vi "Pre Launch Init.vi"(11 "TopLevel in":refnum<class "TopLevel.lvclass">) -> (0 "error out":errorcluster, 3 "TopLevel out":refnum<class "TopLevel.lvclass">)   [LabVIEW 2019, in "TopLevel.lvlib" / "TopLevel.lvclass"]
doc: "(<B>Filename</B>: Actor Framework.lvlib:Actor.lvclass:Pre Launch Init.vi)\n\nDefines behavior that occurs after the Launch Nested Actor method is invoked but before the actor's Actor Core method begins running.\n\nBy default, this method does nothing. A descendant class may override it to define behavior."
uses:
  TopLevel.lvclass
  C:/Program Files/National Instruments/LabVIEW 2019/vi.lib/ActorFramework/Actor/Actor.lvclass
  TopLevel Messages/SendHistoryResults Msg/SendHistoryResults Msg.lvclass
  C:/Program Files/National Instruments/LabVIEW 2019/vi.lib/ActorFramework/Message/Message.lvclass
  Models/ImageResultModel.ctl
  <vilib>/ActorFramework/Actor/Actor.lvclass/Actor.ctl
  <vilib>/ActorFramework/Message Enqueuer/Message Enqueuer.lvclass/Message Enqueuer.ctl
  TopLevel.lvclass/TopLevel.ctl
  <vilib>/ActorFramework/Message Enqueuer/Init from Existing Queue.vi
  <vilib>/ActorFramework/Actor/Actor.lvclass
  <vilib>/ActorFramework/Message Enqueuer/Message Enqueuer.lvclass
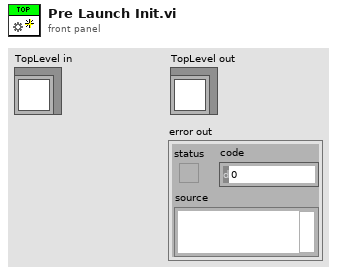
[diagram p1: front panel]
types:
  T1 = typedef "ImageResultModel.ctl" = cluster{"image":string, "pass":bool, "class":string}
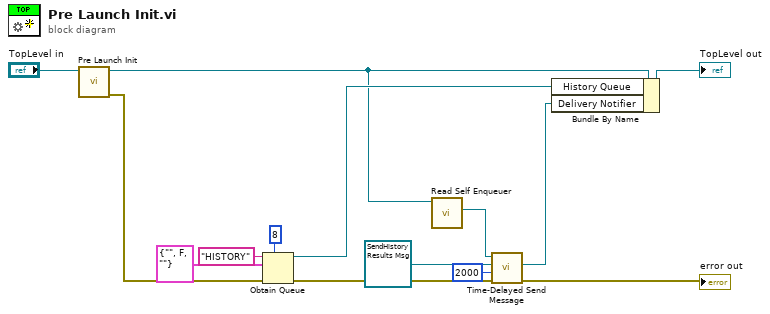
[diagram p0: block diagram]
diagram:
  n1 = call-parent "Pre Launch Init.vi"("Actor in"="TopLevel in") -> ("error out"=w13:errorcluster, "Actor out"=w3:refnum<class "TopLevel.lvclass">)  [unwired: 9 in]
  n2 = Obtain Queue(max queue size (-1, unlimited)=8, name (unnamed)="HISTORY", element data type=T1 {"image"="", "pass"=FALSE, "class"=""} ("Cluster"), error in (no error)=w13) -> (queue out=w9:refnum<queue>, error out=w8:errorcluster)  [unwired: 1 in, 1 out]
  n3 = call <vilib>:"Read Self Enqueuer.vi"("Actor"=w3) -> ("Self Enqueuer"=w5:refnum<class "Message Enqueuer.lvclass">)  [unwired: 10 in]
  n4 = call <vilib>:"Time-Delayed Send Message.vi"("error in (no error)"=w8, "Milliseconds To Wait"=2000, "Message"=refnum<class "SendHistoryResults Msg.lvclass"> refnum ("TopLevel.lvlib:SendHistoryResults Msg.lvclass"), "Message Enqueuer"=w5) -> ("error out"=→"error out":errorcluster, "Delivery Notifier"=w1:refnum<notifier>)  [unwired: 6 in]
  n5 = Bundle By Name(cluster=w3, "History Queue"=w9, "Delivery Notifier"=w1) -> (→"TopLevel out":refnum<class "TopLevel.lvclass">)
